vi "To String.vi"(8 "error in (no error)":errorcluster, 11 "Double Float in":refnum<class "Abs_Complex Extended Float.lvclass">) -> (0 "error out":errorcluster, 2 "String":string, 3 "Double Float out":refnum<class "Abs_Complex Extended Float.lvclass">)   [LabVIEW 2021, in "Abs_Complex Extended Float.lvclass"]
uses:
  Abs_Complex Extended Float.lvclass
  C:/Program Files (x86)/National Instruments/LabVIEW 2021/vi.lib/TSA/Abstract Data Classes/Abs_Types/Numeric/Abs_Numeric.lvclass
  Numeric/Abs_Numeric.lvclass/Abs_Numeric.ctl
  Numeric/Properties/Read Units.vi
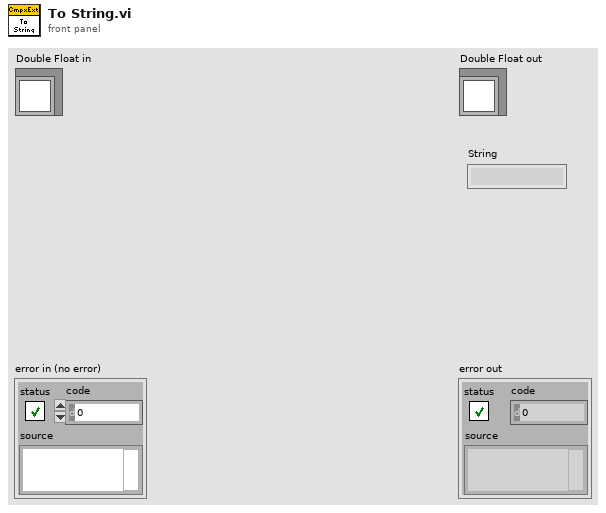
[diagram p1: front panel]
types:
  T1 = typedef "Abs_Complex Extended Float.lvclass/Type.ctl" = cxt
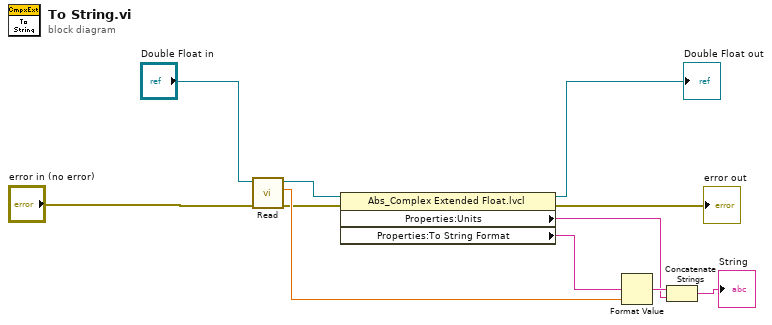
[diagram p0: block diagram]
diagram:
  n1 = call-dynamic "Read.vi"("error in (no error)"="error in (no error)", "Double Float.lvclass_340760 in"="Double Float in") -> ("error out"=w3:errorcluster, "Value"=w4:T1, "Double Float.lvclass_340760 out"=w5:refnum<class "Abs_Complex Extended Float.lvclass">)  [unwired: 7 in]
  n2 = property class="Abs_Complex Extended Float.lvcl"(reference=w5, error in=w3) -> (reference out=→"Double Float out":refnum<class "Abs_Complex Extended Float.lvclass">, error out=→"error out":errorcluster, "Properties:Units"=w1:string, "Properties:To String Format"=w6:string)
  n3 = Format Value(format string=w6, value (0)=w4) -> (output string=w10:string)  [unwired: 1 in]
  n4 = Concatenate Strings(w10, w1) -> (→"String":string)
